vi "Structured Light Codev2.vi"() -> ()   [LabVIEW 2014]
uses:
  <vilib>/userdefined/High Color/IMAQdx.ctl
  <vilib>/vision/driver/NI_Vision_Acquisition_Software.lvlib
panel:
  out "Distance Array\nin inches":dbl[](array[numeric])
  out "Occupancy Grid":dbl[][](graph)
  out "Sorted Particle Measurements":dbl[][](array[numeric]) format="%.2f"
  out "Number of \nSegments Found":i32
  out "Image at Output of Vision Code":T1(plugin-control)
  out "Original Image from Camera":T1(plugin-control)
  in  "stop":bool
  out "Running Light":bool
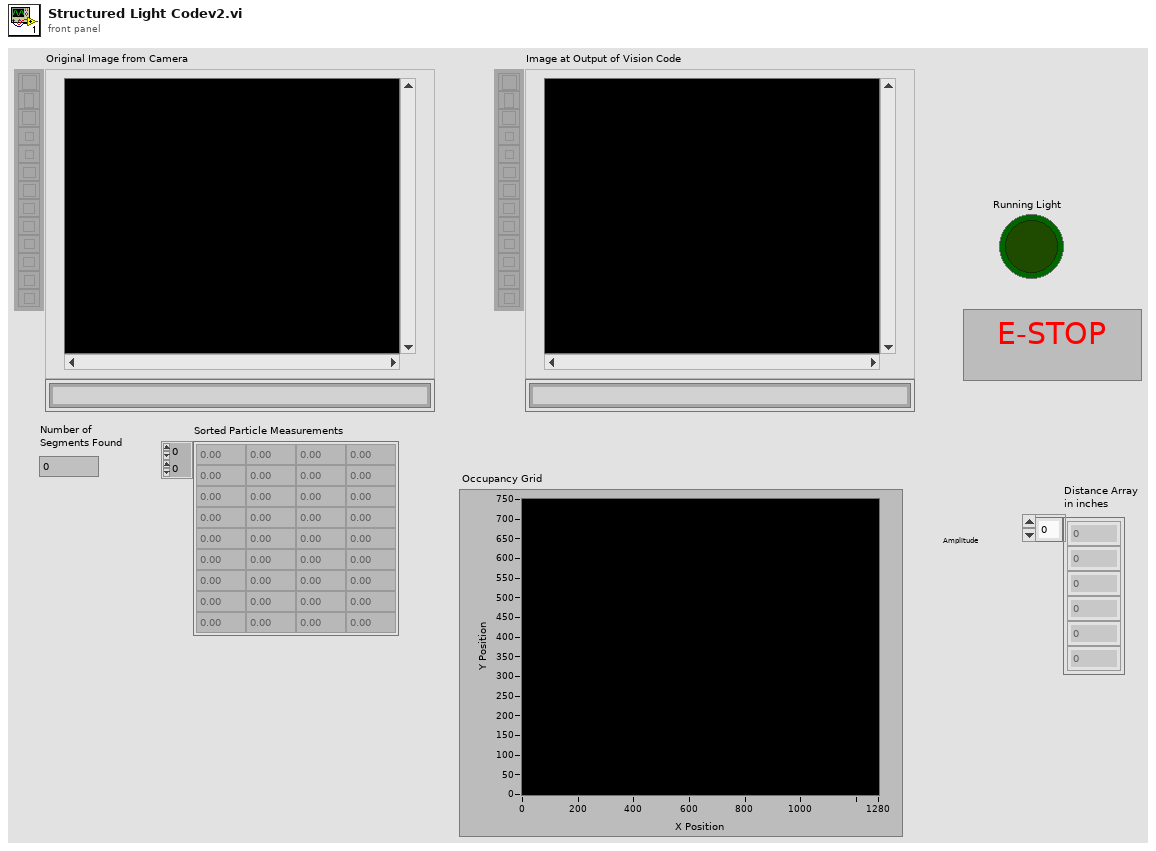
[diagram p1: front panel]
types:
  T1 = typedef "IMAQ Image.ctl" = refnum<image>
  T2 = typedef "IMAQdx.ctl" = refnum<k21>
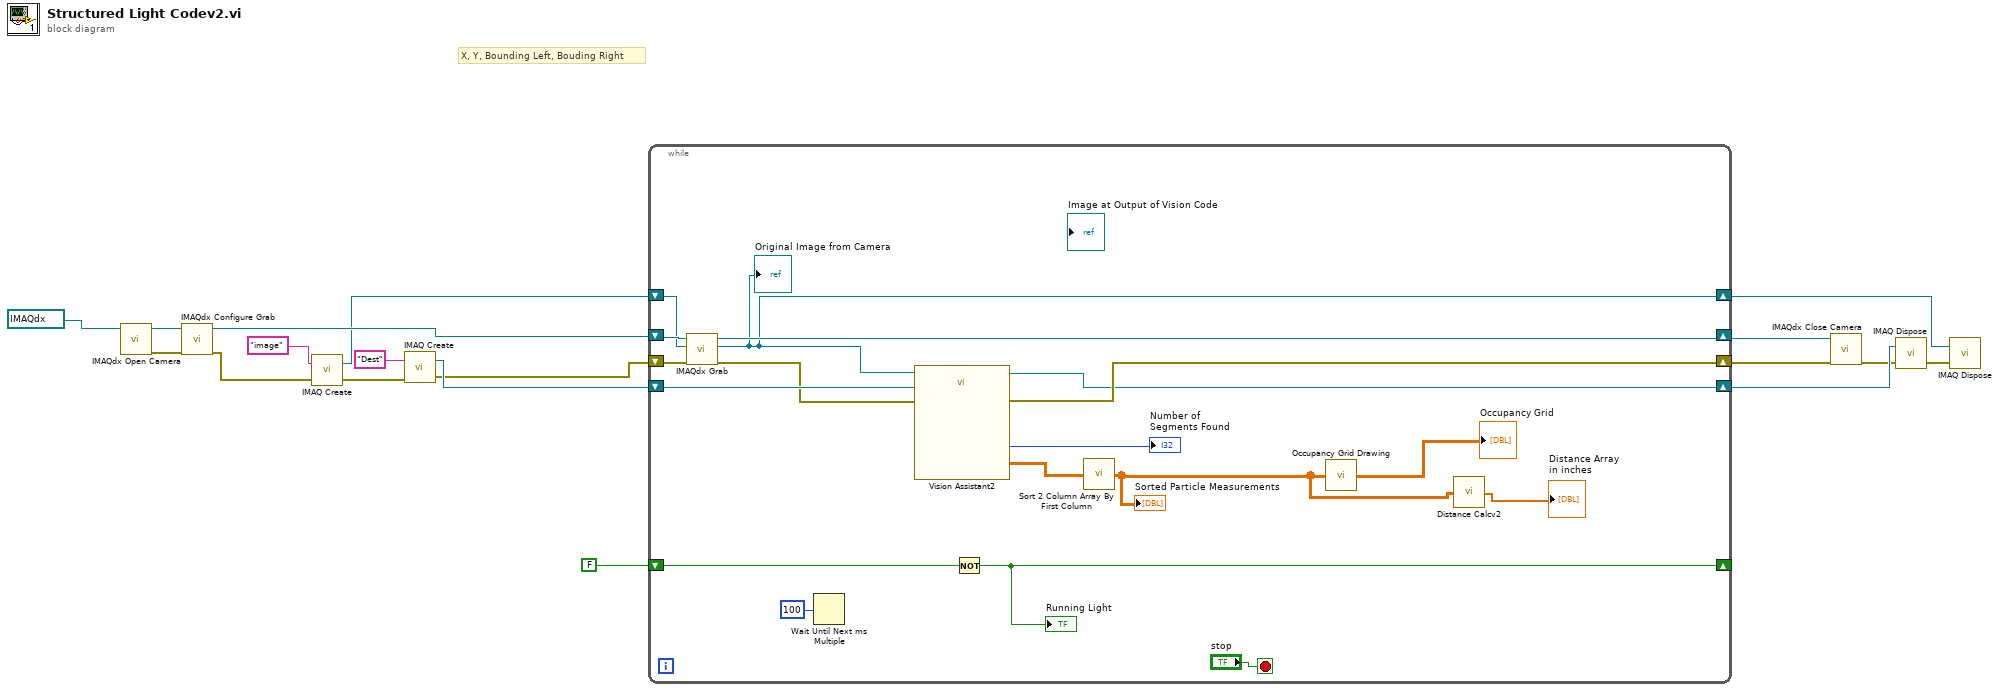
[diagram p0: block diagram]
diagram:
  # "X, Y, Bounding Left, Bouding Right"
  n1 = call <vilib>:"IMAQdx Open Camera.vi"("Session In"=T2 "cam1") -> ("error out"=w17:errorcluster, "Session Out"=w16:T2)  [unwired: 9 in]
  n2 = call <vilib>:"IMAQdx Configure Grab.vi"("error in"=w17, "Session In"=w16) -> ("error out"=w13:errorcluster, "Session Out"=w15:T2)  [unwired: 8 in]
  n3 = call "IMAQ Create"("Image Name"="image", "error in (no error)"=w13) -> ("New Image"=w9:T1, "error out"=w11:errorcluster)  [unwired: 3 in]
  n4 = call "IMAQ Create"("Image Name"="Dest", "error in (no error)"=w11) -> ("New Image"=w8:T1, "error out"=w1:errorcluster)  [unwired: 3 in]
  n5 = while {
    shift-right: [w32] -> _
    shift-left: FALSE -> [w33]
    shift-right: [w25] -> w6
    shift-left: w1 -> [w30]
    shift-right: [w29] -> w7
    shift-left: w15 -> [w36]
    shift-right: [w28] -> w2
    shift-left: w9 -> [w35]
    shift-right: [w24] -> w5
    shift-left: w8 -> [w27]
    stop <- "stop" stop-if-true
    n6 = call <vilib>:"IMAQdx Grab.vi"("error in"=w30, "Image In"=w35, "Session In"=w36) -> ("error out"=w26:errorcluster, "Image Out"=w28:T1, "Session Out"=w29:T2)  [unwired: 5 in, 1 out]
    "Original Image from Camera" <- w28
    n7 = Wait Until Next ms Multiple(millisecond multiple=u32 100) -> ()  [unwired: 1 out]
    n8 = call "Vision Assistant2"("Image In"=w28, "Image Dst"=w27, "error in"=w26) -> ("Image Out"=w24:T1, "Number of Particles (Particle Analysis 1)"=→"Number of \nSegments Found":i32, "Particle Measurements (Pixels) (Particle Analysis 1)"=w22:dbl[][], "error out"=w25:errorcluster)  [unwired: 21 in]
    n9 = Not(x=w33) -> (.not. x?=w32:bool)
    "Running Light" <- w32
    n10 = call "Sort 2 Column Array By First Column.vi"("2D array to sort"=w22) -> ("Sorted array"=w19:dbl[][])
    "Sorted Particle Measurements" <- w19
    n11 = call "Occupancy Grid Drawing.vi"("Particle Points"=w19) -> ("Output Occupancy Grid"=→"Occupancy Grid":dbl[][])
    n12 = call "Distance Calcv2.vi"("Particle Points"=w19) -> ("Output Distance Array"=→"Distance Array\nin inches":dbl[])
  }
  n13 = call <vilib>:"IMAQdx Close Camera.vi"("error in"=w6, "Session In"=w7) -> ("error out"=w4:errorcluster)  [unwired: 9 in]
  n14 = call "IMAQ Dispose"("Image"=w5, "error in (no error)"=w4) -> ("error out"=w3:errorcluster)  [unwired: 4 in]
  n15 = call "IMAQ Dispose"("Image"=w2, "error in (no error)"=w3) -> ()  [unwired: 4 in, 1 out]
